vi "Wrapper.vi"(8 "error in":errorcluster, 11 "Actor in":refnum<class "Actor.lvclass">) -> (0 "error out":errorcluster, 3 "Controller out":refnum<class "Controller.lvclass">)   [LabVIEW 2015, in "Controller.lvlib" / "Stop PAS Wvfm Write MSG.lvclass"]
uses:
  Stop PAS Wvfm Write MSG.lvclass
  Controller.lvclass
  <vilib>/ActorFramework/Message Enqueuer/Message Enqueuer.lvclass
  Controls/eMap.ctl
  <vilib>/ActorFramework/Stop Msg/Stop Msg.lvclass
  reusable/Session APIs/Session Log/System Log.lvclass
  <vilib>/ActorFramework/Actor/Actor.lvclass
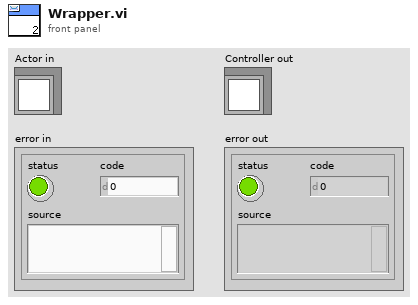
[diagram p1: front panel]
types:
  T1 = typedef "Session - Root.lvclass/Session Handle.ctl" = refnum<data-value>
  T2 = typedef "Controller.lvlib/Controller.lvclass/eMap.ctl" = cluster{"Enqueuer":refnum<class "Message Enqueuer.lvclass">, "Active":bool}
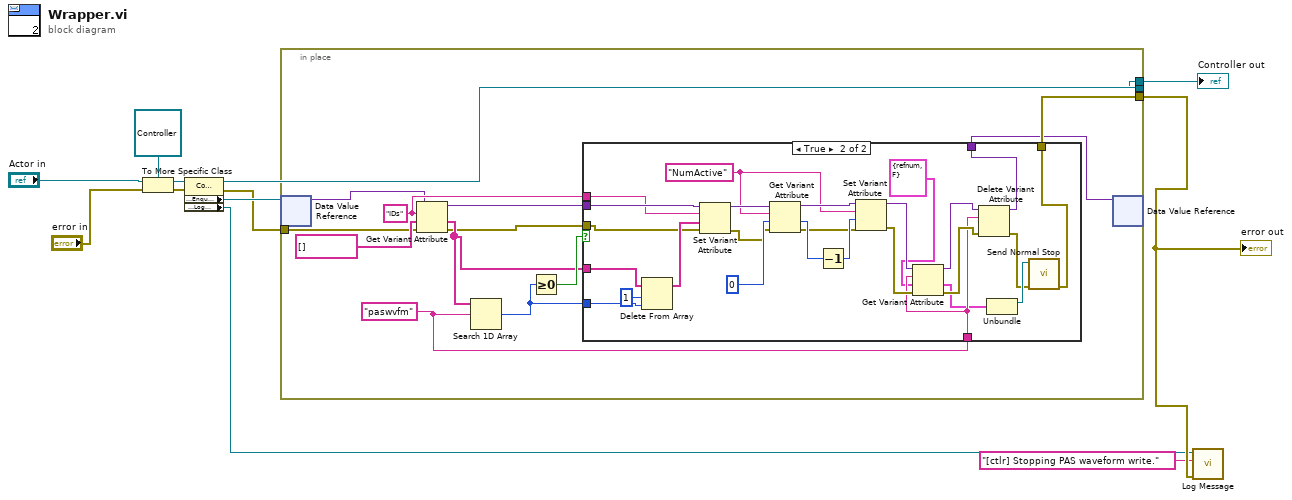
[diagram p0: block diagram]
diagram:
  n1 = To More Specific Class(target class=refnum<class "Controller.lvclass"> refnum ("Controller:Controller"), reference="Actor in", error in="error in") -> (specific class reference=w4:refnum<class "Controller.lvclass">, error out=w5:errorcluster)
  n2 = property class="Controller"(reference=w4, error in=w5) -> (reference out=w7:refnum<class "Controller.lvclass">, error out=w6:errorcluster, "Accessors:Enqueuer MAP DVR"=w9:refnum<data-value>, "Accessors:Log Session"=w10:T1)
  n3 = in-place {
    in-place-border: w6 -> [w18]
    in-place-border: w7 -> [w16]
    in-place-border: [w16] -> w8
    in-place-border: [w15] -> w12
    w17 = "paswvfm" ("element")
    w20 = "IDs" ("name")
    n4 = in-place-dvr #1(w9) -> (w14:variant)  [unwired: 1 out]
    n5 = Get Variant Attribute(Variant=w14, name=w20, default value (empty Variant)=string[] [], error in=w18) -> (duplicate Variant=w24:variant, value=w21:string[], error out=w19:errorcluster)  [unwired: 1 out]
    n6 = Search 1D Array(1D array=w21, element=w17) -> (index of element=w22:i32)  [unwired: 1 in]
    n7 = Greater Or Equal To 0?(x=w22) -> (x >= 0?=w23:bool)
    n8 = case shown="True" w23 {
      tunnel: w24 -> [w26 w53]
      tunnel: w22 -> [_ w52]
      tunnel: w21 -> [_ w50]
      tunnel: w20 -> [_ w48]
      tunnel: w19 -> [w27 w39]
      tunnel: w17 -> [_ w33]
      tunnel: [w26 w38] -> w13
      tunnel: [w27 w28] -> w15
      frame False {
      }
      frame True {
        w42 = "NumActive" ("name")
        n9 = Delete From Array(array=w50, length=1, index=w52) -> (array with subset deleted=w49:string[])  [unwired: 1 out]
        n10 = Set Variant Attribute(Variant=w53, name=w48, value=w49, error in=w39) -> (Variant out=w47:variant, error out=w40:errorcluster)  [unwired: 1 out]
        n11 = Get Variant Attribute(Variant=w47, name=w42, default value (empty Variant)=i16 0, error in=w40) -> (duplicate Variant=w43:variant, value=w45:i16, error out=w41:errorcluster)  [unwired: 1 out]
        n12 = Decrement(x=w45) -> (x-1=w44:i16)
        n13 = Set Variant Attribute(Variant=w43, name=w42, value=w44, error in=w41) -> (Variant out=w37:variant, error out=w34:errorcluster)  [unwired: 1 out]
        n14 = Get Variant Attribute(Variant=w37, name=w33, default value (empty Variant)=T2 {"Enqueuer"=refnum, "Active"=FALSE} ("eMap"), error in=w34) -> (duplicate Variant=w36:variant, value=w31:T2, error out=w35:errorcluster)  [unwired: 1 out]
        n15 = Delete Variant Attribute(4:w35, 6:w33, 7:w36) -> (0:w29:errorcluster, 3:w38:variant)  [unwired: 1 out]
        n16 = Unbundle(w31) -> ("Enqueuer"=w30:refnum<class "Message Enqueuer.lvclass">)  [unwired: 1 out]
        n17 = call <vilib>:"Send Normal Stop.vi"("error in (no error)"=w29, "Message Enqueuer"=w30) -> ("error out"=w28:errorcluster)  [unwired: 9 in]
      }
    }
    n18 = in-place-dvr #1(w13) -> ()  [unwired: 2 out]
  }
  "error out" <- w12
  "Controller out" <- w8
  n19 = call "Log Message.vi"("error in"=w12, "MSG In"="[ctlr] Stopping PAS waveform write.", "session in"=w10) -> ()  [unwired: 7 in, 2 out]
